vi "Streamed to Waveform Array Converter.vi"() -> ()   [LabVIEW 2013]
doc: "Use this template to build a user interface event handler design pattern. Use this pattern for dialog boxes and other user interfaces. You also can create and execute user-defined events that the VI can handle the same way as user interface events."
panel:
  out "Streamed Data":dbl[][](graph)
  out "Waveform Data":waveform(dbl)[](graph)
  out "Output Path":path
  out "Record Count":u32
  in  "Sampling Rate":u32=500000
  in  "Record Channel Size":bool
  in  "Path":path
  in  "Convert":bool
  in  "stop":bool
  # "51200"
  # "51200 x 3"
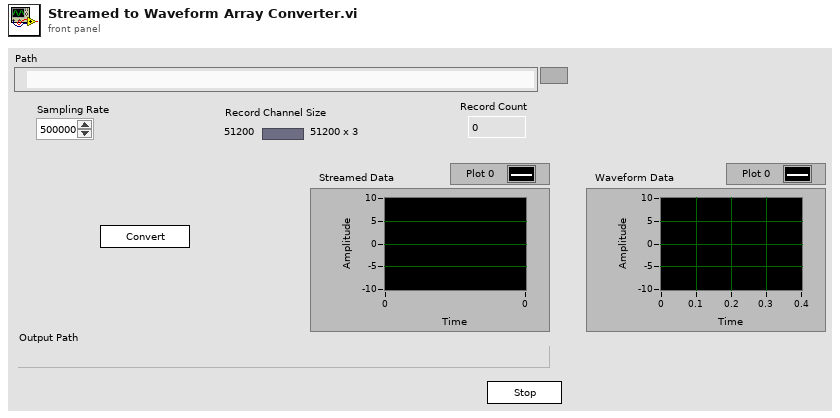
[diagram p1: front panel]
types:
  T1 = enum16{"big-endian, network order", "native, host order", "little-endian"}
  T2 = enum16{"open", "replace", "create", "open or create", "replace or create", "replace or create with confirmation"}
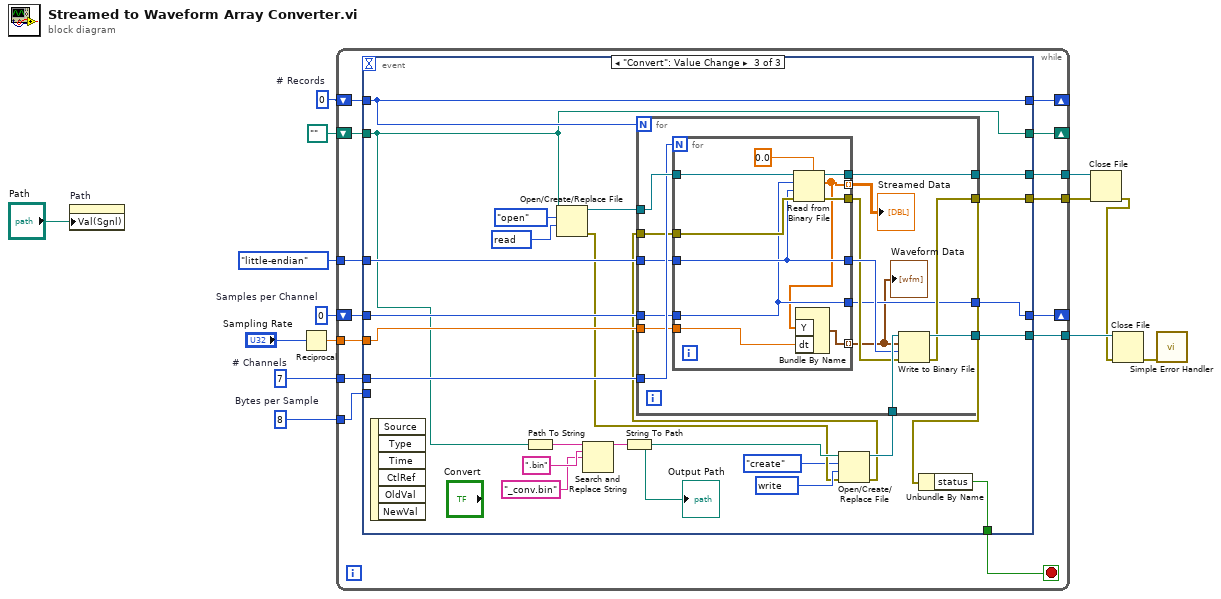
[diagram p0: block diagram]
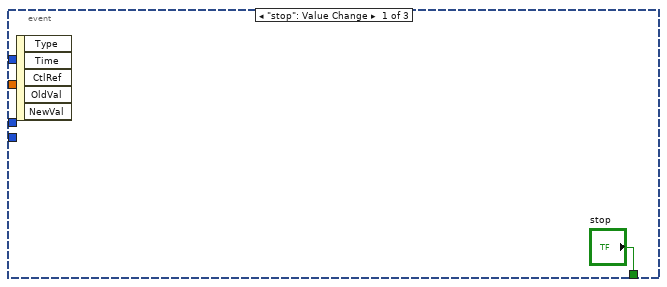
[diagram p2: hidden frame]
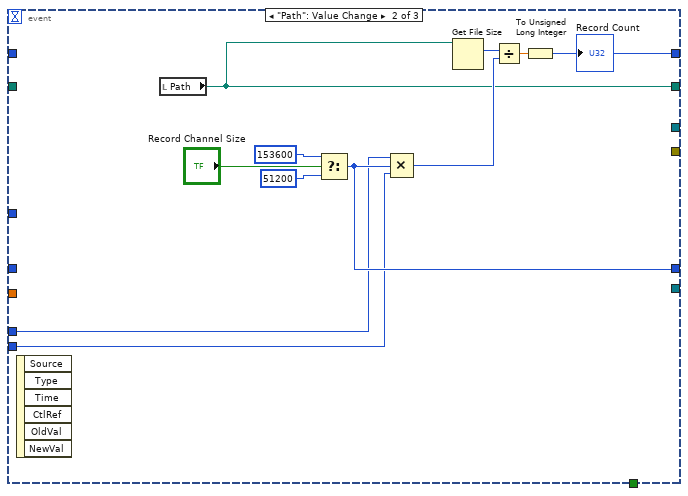
[diagram p3: hidden frame]
diagram:
  w10 = u32 8  # Bytes per Sample
  w11 = u32 7  # # Channels
  w12 = u32 0  # Samples per Channel
  w14 = u32 0  # # Records
  n1 = property on="Path" class="Path"("Val(Sgnl)"="Path") -> ()  [unwired: 2 in, 2 out]
  n2 = Reciprocal(x="Sampling Rate") -> (1/x=w8:dbl)
  n3 = while {
    shift-right: [w27] -> _
    shift-left: w14 -> [w26]
    shift-right: [w25] -> _
    shift-left: path "" ("Path") -> [w24]
    shift-right: [w23] -> _
    shift-left: w12 -> [w22]
    tunnel: w11 -> [w21]
    tunnel: w10 -> [w20]
    tunnel: w8 -> [w19]
    tunnel: T1."little-endian" ("byte order (0:big-endian, network order)") -> [w18]
    tunnel: [w17] -> w5
    tunnel: [w16] -> w6
    tunnel: [w15] -> w4
    stop <- w28 stop-if-true
    n4 = event shown="[2] \"Convert\": Value Change" {
      selector: _ -> [_ _ _]
      dyn-events: _ -> [_ _ _]
      timeout: _ -> [_ _ _]
      tunnel: ["stop" _ w41] -> w28
      tunnel: [_ w39 w47] -> w27
      tunnel: w26 -> [_ _ w47]
      tunnel: [_ w32 w46] -> w25
      tunnel: w24 -> [_ _ w46]
      tunnel: [_ w35 w45] -> w23
      tunnel: w22 -> [_ _ w55]
      tunnel: w21 -> [_ w34 w56]
      tunnel: w20 -> [_ w33 _]
      tunnel: w19 -> [_ _ w54]
      tunnel: w18 -> [_ _ w53]
      tunnel: [_ _ w51] -> w17
      tunnel: [_ _ w50] -> w16
      tunnel: [_ _ w42] -> w15
      event "stop": Value Change {
        n5 = event-data() -> ()  [unwired: 1 in, 5 out]
      }
      event "Path": Value Change {
        n6 = event-data() -> ()  [unwired: 1 in, 6 out]
        n7 = local read "Path"() -> (w32:path)
        n8 = Select(t=u32 153600, s="Record Channel Size", f=u32 51200) -> (s? t:f=w35:u32)
        n9 = Compound Arithmetic op=MULTIPLY(w34, w35, w33) -> (w36:u32)
        n10 = Get File Size(file=w32) -> (size (in bytes)=w37:i64)  [unwired: 1 in, 2 out]
        n11 = Divide(x=w37, y=w36) -> (x/y=w38:dbl)
        n12 = To Unsigned Long Integer(number=w38) -> (unsigned 32bit integer=w39:u32)
        "Record Count" <- w39
      }
      event "Convert": Value Change {
        w59 = u32 1073741824 items=["read"=2147483648, "write"=1073741824, "read & write"=3221225472, "execute"=536870912, "all"=268435456] ("desired access (read & write)")
        w64 = u32 2147483648 items=["read"=2147483648, "write"=1073741824, "read & write"=3221225472, "execute"=536870912, "all"=268435456] ("desired access (read & write)")
        n13 = event-data() -> ()  [unwired: 1 in, 6 out]
        n14 = Path To String(path=w46) -> (string=w63:string)
        n15 = Open/Create/Replace File(file path (use dialog)=w46, operation (0:open)=T2."open", access (0:read/write)=w64) -> (refnum out=w57:refnum<file>, error out=w49:errorcluster)  [unwired: 3 in, 1 out]
        n16 = Search and Replace String(input string=w63, search string=".bin", replace string="_conv.bin" ("replace string (\"\")")) -> (result string=w60:string)  [unwired: 5 in, 3 out]
        n17 = String To Path(string=w60) -> (path=w58:path)
        "Output Path" <- w58
        n18 = Open/Create/Replace File(file path (use dialog)=w58, error in=w49, operation (0:open)=T2."create", access (0:read/write)=w59) -> (refnum out=w52:refnum<file>, error out=w48:errorcluster)  [unwired: 2 in, 1 out]
        n19 = for {
          N: w47 -> [_]
          tunnel: w57 -> [w79]
          tunnel: w56 -> [w78]
          tunnel: w55 -> [w77]
          tunnel: w48 -> [w76]
          tunnel: w54 -> [w75]
          tunnel: w53 -> [w74]
          tunnel: w52 -> [w73]
          tunnel: [w70] -> w51
          tunnel: [w69] -> w50
          tunnel: [w68] -> w42
          tunnel: [w67] -> w45
          n20 = for {
            N: w78 -> [_]
            tunnel: [w89] -> w66 mode=indexing
            tunnel: w79 -> [w87]
            tunnel: w77 -> [w81]
            tunnel: w76 -> [w86]
            tunnel: w75 -> [w85]
            tunnel: w74 -> [w83]
            tunnel: [w84] -> w71
            tunnel: [w83] -> w72
            tunnel: [w82] -> w69
            tunnel: [w81] -> w67
            tunnel: [w80] -> w65 mode=indexing
            n21 = Read from Binary File(5:0.0, 8:w86, 9:w83, 10:w81, 11:w87) -> (0:w84:errorcluster, 2:w80:dbl[], 3:w82:refnum<file>)  [unwired: 1 in, 1 out]
            n22 = Bundle By Name("Y"=w80, "dt"=w85) -> (w89:waveform(dbl))  [unwired: 1 in]
          }
          "Waveform Data" <- w66
          "Streamed Data" <- w65
          n23 = Write to Binary File(file (use dialog)=w73, data=w66, error in=w71, 9:w72) -> (refnum out=w70:refnum<file>, error out=w68:errorcluster)  [unwired: 2 in, 1 out]
        }
        n24 = Unbundle By Name(w42) -> ("status"=w41:bool)
      }
    }
  }
  n25 = Close File(refnum=w6, error in=w4) -> (error out=w3:errorcluster)  [unwired: 1 out]
  n26 = Close File(refnum=w5, error in=w3) -> (error out=w1:errorcluster)  [unwired: 1 out]
  n27 = call <vilib>:"Simple Error Handler.vi"("error in (no error)"=w1) -> ()  [unwired: 4 in, 5 out]
